vi "Read Desired Temperature.vi"(11 "冷却器输入":refnum<class "Cooler.lvclass">) -> (2 "待维持的温度":dbl=75.0)   [LabVIEW 2013, in "Cooler.lvlib" / "Cooler.lvclass"]
doc: "读取系统需要维持的温度。"
uses:
  Cooler.lvclass
  Level Controller/Level Controller/Level Controller.lvclass
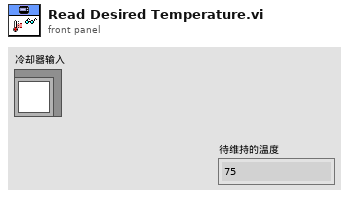
[diagram p1: front panel]
types:
  T1 = typedef "Level Controller.lvlib/Level Controller.lvclass/Deadband.ctl" = cluster{"Low":dbl, "High":dbl}
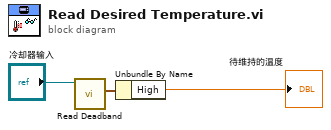
[diagram p0: block diagram]
diagram:
  n1 = call "Read Deadband.vi"("水位控制器输入"="冷却器输入") -> ("死区"=w2:T1)  [unwired: 8 in, 2 out]
  n2 = Unbundle By Name(w2) -> ("High"=→"待维持的温度":dbl)
